vi "Untitled 1.vi"(8 "error in (no error)":errorcluster, 11 "NeedleValve in":refnum<class "NeedleValve.lvclass">) -> (0 "error out":errorcluster, 2 "Angele":dbl, 3 "NeedleValve out":refnum<class "NeedleValve.lvclass">)   [LabVIEW 2019, in "NeedleValve.lvclass"]
uses:
  NeedleValve.lvclass
  NeedleValve.lvclass/NeedleValve.ctl
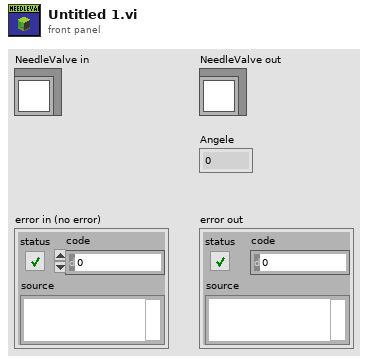
[diagram p1: front panel]
types:
  T1 = typedef "Needle Valve Data.ctl" = cluster{"Engine State":T2, "StateValveModbus":T3, "Alarms":T4, "RAW":i32, "Angele":dbl, "Step":i32, "Encoder":i32, "Kinematic":T5, "Limits":T6, "EncoderMax":i32, "Counter Max Dont Update":i32, "EncoderMin":i32, "Counter Min Dont Update":i32, "Prepere Counter":i32, "STEP INIT":i32, "offset - Angel":dbl}
  T2 = typedef "MB_ENGINE.lvclass/Engine State.ctl" = u16
  T3 = typedef "Needle Valve State.ctl" = enum16{"STOPED", "CLOSED", "OPENED", "OPENING", "CLOSING", "FULL_CLOSE", "PREP_OPEN"}
  T4 = typedef "MB_ENGINE.lvclass/Engine Alarms.ctl" = cluster{"OL":bool, "TF":bool, "STL":bool, "OCP":bool, "CPUV":bool, "UVLO":bool, "SPI_ERROR":bool, "Fault":bool, "OL 2":bool, "TF 2":bool, "STL 2":bool, "OCP 2":bool, "CPUV 2":bool, "UVLO 2":bool, "reserved":bool, "InitDone":bool}
  T5 = typedef "MB_ENGINE.lvclass/Settings.ctl" = cluster{"ACC Steps Per Sec^2":u16, "DEC Steps Per Sec^2":u16, "Min Velosity Step Per Sec":u16, "Max Velosity Step Per Sec":u16, "MicroStep":u16}
  T6 = typedef "MB_ENGINE.lvclass/Limits Status.ctl" = cluster{"Fault 2 Switch":bool, "Fault 1 Switch":bool, "Center(Home)":bool, "Lower Limit":bool, "Upper Limit":bool}
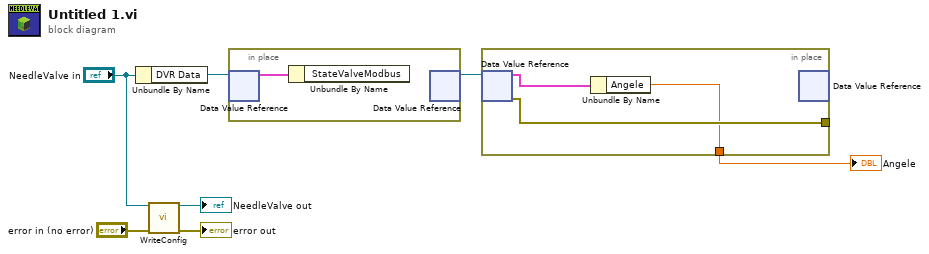
[diagram p0: block diagram]
diagram:
  n1 = Unbundle By Name("NeedleValve in") -> ("DVR Data"=w6:refnum<data-value>)
  n2 = call-dynamic "WriteConfig.vi"("reference in"="NeedleValve in", "error in (no error)"="error in (no error)") -> ("reference out"=→"NeedleValve out":refnum<class "NeedleValve.lvclass">, "error out"=→"error out":errorcluster)  [unwired: 12 in]
  n3 = in-place {
    n4 = in-place-dvr #1(w6) -> (w8:T1)  [unwired: 1 out]
    n5 = Unbundle By Name(w8) -> ()  [unwired: 1 out]
    n6 = in-place-dvr #1() -> (w7:refnum<data-value>)  [unwired: 1 in, 1 out]
  }
  n7 = in-place {
    in-place-border: [w11] -> _
    in-place-border: [w9] -> w5
    n8 = in-place-dvr #2(w7) -> (w10:T1, w11:errorcluster)
    n9 = Unbundle By Name(w10) -> ("Angele"=w9:dbl)
    n10 = in-place-dvr #2() -> ()  [unwired: 1 in, 2 out]
  }
  "Angele" <- w5
